vi "Build all.vi"() -> ()   [LabVIEW 2021]
panel:
  out "Build time":dbl
  out "error out":errorcluster
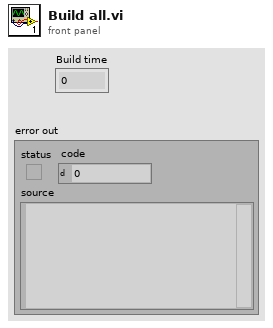
[diagram p1: front panel]
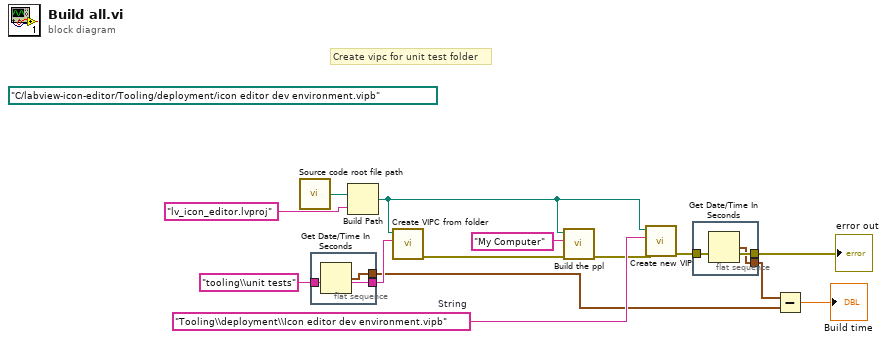
[diagram p0: block diagram]
diagram:
  w14 = "Tooling\\deployment\\Icon editor dev environment.vipb"  # String
  (unwired) path "C:/labview-icon-editor/Tooling/deployment/icon editor dev environment.vipb" ("Project path")
  # "Create vipc for unit test folder"
  n1 = call "Source code root file path.vi"() -> ("Source code root path"=w13:path)  [unwired: 1 in]
  n2 = flat-sequence {
    tunnel: "tooling\\unit tests" ("Dependency folder relative path") -> [w16]
    tunnel: [w16] -> w6
    tunnel: [w15] -> w2
    frame #0 {
      n3 = Get Date/Time In Seconds() -> (seconds since 1Jan1904=w15:timestamp)
    }
  }
  n4 = Build Path(base path=w13, name or relative path="lv_icon_editor.lvproj" ("Dependency folder relative path")) -> (appended path=w10:path)
  n5 = call "Create VIPC from folder.vi"("Dependency folder relative path"=w6, "Project path"=w10) -> ("error out"=w11:errorcluster)  [unwired: 9 in]
  n6 = call "Build the ppl.vi"("error in (no error)"=w11, "Name of target (My Computer)"="My Computer", "Path override"=w10) -> ("error out"=w9:errorcluster)  [unwired: 7 in, 1 out]
  n7 = call "Create new VIP.vi"("error in (no error)"=w9, "String"=w14, "Project path"=w10) -> ("error out"=w5:errorcluster)  [unwired: 7 in, 1 out]
  n8 = flat-sequence {
    tunnel: w5 -> [w18]
    tunnel: [w18] -> w4
    tunnel: [w17] -> w3
    frame #0 {
      n9 = Get Date/Time In Seconds() -> (seconds since 1Jan1904=w17:timestamp)
    }
  }
  n10 = Subtract(x=w3, y=w2) -> (x-y=→"Build time":dbl)
  "error out" <- w4
